vi "Agilent SNA Set Number of Points.vi"(6 "Channel":i8=1 min=1 max=99 step=1, 7 "Agilent SNA & SWP":T1, 8 "error in (no error)":errorcluster, 10 "Number Points":i32, 11 "VISA Resource Names":T2) -> (0 "error out":errorcluster, 3 "dup VISA Resource Names":T2)   [LabVIEW 2011]
doc: "This VI for the HP 8753B is used to read the number of stimulus points."
uses:
  TypeDefs/Agilent SNA VISA.ctl
  TypeDefs/Agilent SNA Instrument Info.ctl
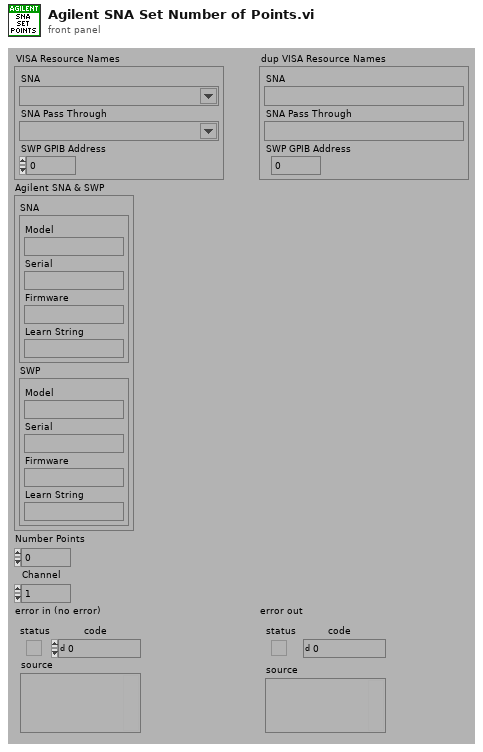
[diagram p1: front panel]
types:
  T1 = typedef "Agilent SNA Instrument Info.ctl" = cluster{"SNA":cluster{"Model":string, "Serial":string, "Firmware":string, "Learn String":string}, "SWP":cluster{"Model":string, "Serial":string, "Firmware":string, "Learn String":string}}
  T2 = typedef "Agilent SNA VISA.ctl" = cluster{"SNA":refnum<visa-resource-name>, "SNA Pass Through":refnum<visa-resource-name>, "SWP GPIB Address":i32}
  T3 = typedef "Agilent SNA Model.ctl" = enum16{"Not Supported", "8757X"}
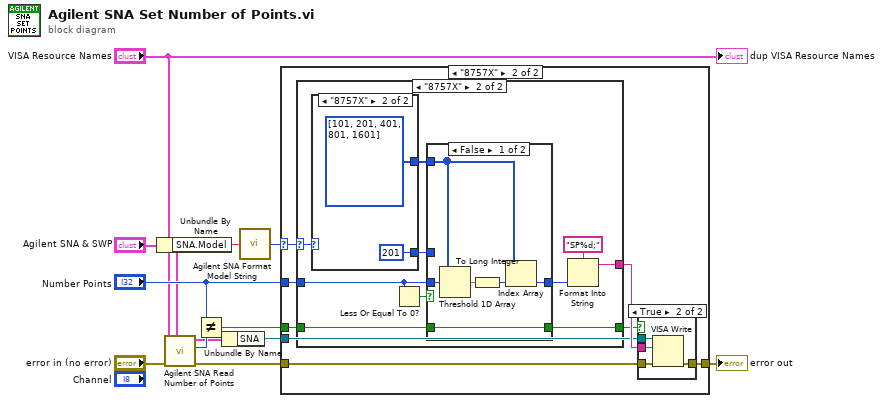
[diagram p0: block diagram]
diagram:
  n1 = Unbundle By Name("Agilent SNA & SWP") -> ("SNA.Model"=w4:string)
  n2 = call "Agilent SNA Read Number of Points.vi"("Agilent SNA & SWP"="Agilent SNA & SWP", "error in (no error)"="error in (no error)", "VISA Resource Names"="VISA Resource Names") -> ("error out"=w8:errorcluster, "Number Points"=w7:i32, "dup VISA Resource Names"=w2:T2)  [unwired: 1 in, 5 out]
  n3 = Not Equal?(x="Number Points", y=w7) -> (x != y?=w10:bool)
  n4 = Unbundle By Name(w2) -> ("SNA"=w1:refnum<visa-resource-name>)
  n5 = call "Agilent SNA Format Model String.vi"("Model String"=w4) -> ("Model"=w5:T3)
  n6 = case shown="\"8757X\"" w5 {
    selector: w5 -> [_ w16]
    tunnel: [w13 w21] -> w12
    tunnel: "Number Points" -> [_ w19]
    tunnel: w10 -> [_ w15]
    tunnel: w1 -> [_ w18]
    tunnel: w8 -> [w13 w17]
    frame "Not Supported" {
    }
    frame "8757X" {
      n7 = case shown="\"8757X\"" w16 {
        selector: w16 -> [_ w24]
        tunnel: [_ w28] -> w20
        tunnel: w19 -> [_ w25]
        tunnel: w15 -> [_ w23]
        tunnel: [_ w22] -> w14
        frame "Not Supported" {
        }
        frame "8757X" {
          n8 = case shown="\"8757X\"" w24 {
            tunnel: [_ i32[] [101, 201, 401, 801, 1601]] -> w30
            tunnel: [_ 201] -> w26
            frame "Not Supported" {
            }
            frame "8757X" {
            }
          }
          n9 = Less Or Equal To 0?(x=w25) -> (x <= 0?=w27:bool)
          n10 = case shown="False" w27 {
            selector: w27 -> [_ w38]
            tunnel: w30 -> [w36 _]
            tunnel: [w34 w39] -> w29
            tunnel: w25 -> [w33 _]
            tunnel: w26 -> [_ w39]
            tunnel: w23 -> [w32 _]
            tunnel: [w32 w38] -> w22
            frame False {
              n11 = Threshold 1D Array(2:w33, 3:w36) -> (0:w37:dbl)  [unwired: 1 out]
              n12 = To Long Integer(number=w37) -> (32bit integer=w35:i32)
              n13 = Index Array(array=w36, index=w35) -> (element=w34:i32)
            }
            frame True {
            }
          }
          n14 = Format Into String(format string="SP%d;", w29) -> (resulting string=w28:string)  [unwired: 2 in, 1 out]
        }
      }
      n15 = case shown="True" w14 {
        tunnel: w18 -> [_ w46]
        tunnel: w17 -> [w42 w45]
        tunnel: [w42 w44] -> w21
        tunnel: w20 -> [_ w43]
        frame False {
        }
        frame True {
          n16 = VISA Write(VISA resource name=w46, write buffer=w43, error in (no error)=w45) -> (error out=w44:errorcluster)  [unwired: 2 out]
        }
      }
    }
  }
  "error out" <- w12
  "dup VISA Resource Names" <- "VISA Resource Names"
